vi "Find Tagged Object.vi"(7 "RegExp Search?":bool, 8 "error in (no error)":errorcluster, 9 "TagValue":string, 10 "TagName":string="phygbuTag", 11 "Array of References":refnum<vi>[](array[refnum])) -> (0 "error out":errorcluster, 2 "Found?":bool, 3 "reference":refnum<vi>)   [LabVIEW 2012, in "Scripting Tools.lvlib"]
doc: "Searches all the references in Array of references for one that is tagged with the given tag and value."
uses:
  Scripting Tools.lvlib
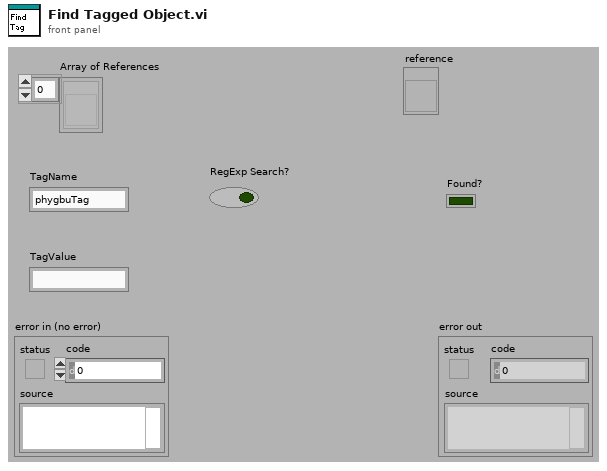
[diagram p1: front panel]
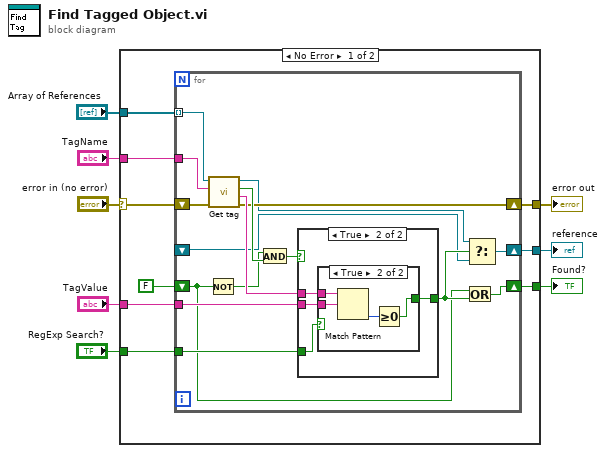
[diagram p0: block diagram]
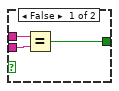
[diagram p3: hidden frame]
diagram:
  n1 = case shown="No Error" "error in (no error)" {
    selector: "error in (no error)" -> [w16 w45]
    tunnel: "Array of References" -> [w17 _]
    tunnel: "TagName" -> [w15 _]
    tunnel: "RegExp Search?" -> [w13 _]
    tunnel: "TagValue" -> [w12 _]
    tunnel: [w11 w45] -> w1
    tunnel: [w10 _] -> w3
    tunnel: [w9 _] -> w2
    frame No Error {
      n2 = for {
        tunnel: w17 -> [w31] mode=indexing
        shift-right: [w19] -> w9
        shift-left: FALSE -> [w18]
        shift-right: [w24] -> w11
        shift-left: w16 -> [w33]
        tunnel: w15 -> [w32]
        tunnel: w13 -> [w29]
        tunnel: w12 -> [w27]
        shift-right: [w20] -> w10
        shift-left: _ -> [w21]
        n3 = Not(x=w18) -> (.not. x?=w25:bool)
        n4 = call "Get tag.vi"("error in (no error)"=w33, "TagName"=w32, "reference"=w31) -> ("error out"=w24:errorcluster, "Tag Value"=w28:string, "Tag Found ?"=w30:bool, "reference Out"=w22:refnum<vi>)  [unwired: 5 out]
        n5 = And(x=w25, y=w30) -> (x .and. y?=w26:bool)
        n6 = case shown="True" w26 {
          tunnel: w29 -> [_ w37]
          tunnel: w28 -> [_ w36]
          tunnel: w27 -> [_ w35]
          tunnel: [_ w34] -> w23
          frame False {
          }
          frame True {
            n7 = case shown="True" w37 {
              tunnel: w36 -> [w40 w44]
              tunnel: w35 -> [w39 w43]
              tunnel: [w38 w41] -> w34
              frame False {
                n8 = Equal?(x=w40, y=w39) -> (x = y?=w38:bool)
              }
              frame True {
                n9 = Match Pattern(string=w44, regular expression=w43) -> (offset past match=w42:i32)  [unwired: 4 out]
                n10 = Greater Or Equal To 0?(x=w42) -> (x >= 0?=w41:bool)
              }
            }
          }
        }
        n11 = Or(x=w18, y=w23) -> (x .or. y?=w19:bool)
        n12 = Select(t=w22, s=w23, f=w21) -> (s? t:f=w20:refnum<vi>)
      }
    }
    frame Error {
    }
  }
  "reference" <- w3
  "error out" <- w1
  "Found?" <- w2
